vi "Test App Remove Process.vi"(8 "error in (no error)":errorcluster, 11 "Rig Test in":refnum<class "Application Test.lvclass">) -> (0 "error out":errorcluster, 3 "Rig Test out":refnum<class "Application Test.lvclass">)   [LabVIEW 2020, in "Application Test.lvclass"]
uses:
  Application Test.lvclass
  C:/Program Files (x86)/National Instruments/LabVIEW 2020/vi.lib/Astemes/LUnit/Test Case.lvclass
  Framework/Process/Process.lvclass
  Framework/Process/Process.lvclass/Process.ctl
  Framework/Application/Application.lvclass/Application.ctl
  <vilib>/Astemes/LUnit/Test Case.lvclass/Test Case.ctl
  <vilib>/Astemes/LUnit/LUnit Assertion Result.lvclass/LUnit Assertion Result.ctl
  <vilib>/Astemes/LUnit/LUnit Test Case Result.lvclass/LUnit Test Case Result.ctl
  <vilib>/Astemes/LUnit/LUnit Method Result.lvclass/LUnit Method Result.ctl
  Framework/Process/Public/Lifecycle/Get Lifecycle State.vi
  Framework/Process/Protected/Messaging/Request Message.vi
  Framework/Application/Private/Add Process to Map.vi
  Framework/Application/Private/Start Idle Processes if Running.vi
  Framework/Application/Private/Throw Error If Process Already in App.vi
  Framework/Process/Protected/Messaging/Enqueue Message.vi
  Framework/Process/Protected/SubVIs/Set Context.vi
  Framework/Application/Private/Remove Process from App.vi
  Framework/Application/Private/Parse Process Name.vi
  Framework/Application/Private/Remove Process from Map.vi
  Framework/Process/Protected/SubVIs/Clear Context.vi
  <vilib>/Astemes/LUnit/Palette/Pass If Equal.vi/cbf50e99-f124-4847-863a-8e9794d3dede.vi
  Framework/Process/Private/SubVIs/Wait for finish.vi
  Framework/Process/Private/SubVIs/Set Lifecycle State.vi
  <vilib>/Utility/error.llb/Clear Errors.vi
  Framework/Process/Private/SubVIs/Handle Debug Data.vi
  Framework/Process/Private/SubVIs/Enqueue Request Message.vi
  Framework/Application/Public/Get Process.vi
  Framework/Process/Public/Lifecycle/Leave Process Loop.vi
  <vilib>/AdvancedString/Delimited String to 1D String Array.vi
  <vilib>/Astemes/LUnit/Palette/Pass.vi
  <vilib>/Astemes/LUnit/Palette/Fail.vi
  <vilib>/Astemes/LUnit/Compare Variants.vi
  <vilib>/Astemes/LUnit/Describe Comparison.vi
  <vilib>/Astemes/LUnit/Set Assertion Type.vi
  Framework/Logging/Log Debug.vi
  <vilib>/AdvancedString/1D String Array to Delimited String.vi
  <vilib>/Utility/High Resolution Relative Seconds.vi
  Framework/Application/Private/Retrieve Process from App.vi
  Framework/Application/Private/Get Process from Map.vi
  <vilib>/Astemes/LUnit/Add test result.vi
  <vilib>/Astemes/LUnit/LUnit Write Passed.vi
  <vilib>/Astemes/LUnit/LUnit Write Message.vi
  <vilib>/Astemes/LUnit/LUnit Write Description.vi
  <vilib>/Astemes/LUnit/Variant to string.vi
  <vilib>/Astemes/LUnit/LUnit Write Assertion Type.vi
  <vilib>/Astemes/LUnit/LUnit Record Assertion Result.vi
  <vilib>/Astemes/LUnit/LUnit Aggregate Assertion Results.vi
  <vilib>/Astemes/LUnit/Assertion Result/LUnit Read Status.vi
  <vilib>/Astemes/LUnit/LUnit Read Message.vi
  <vilib>/Astemes/LUnit/LUnit Read Description.vi
  <vilib>/Astemes/LUnit/Method Result/LUnit Merge Status.vi
  <vilib>/Astemes/LUnit/LUnit Concatenate result strings.vi
  Framework/Application/Application.lvclass
  C:/Git/astemes-triarc-framework/source/Framework/Process/Process.lvclass
  <vilib>/Utility/error.llb/Error Cluster From Error Code.vi
  Framework/Process/Public/Read Name.vi
  Framework/Process/Private/SubVIs/Wait for Response Message.vi
  <vilib>/Utility/Data Type/Get Type Information.vi
  <vilib>/Utility/LVClass/Get LV Class Name.vi
  <vilib>/Astemes/LUnit/LUnit Assertion Result.lvclass
  Application Test.lvclass/Application Test.ctl
  <vilib>/Astemes/LUnit/Test Case.lvclass
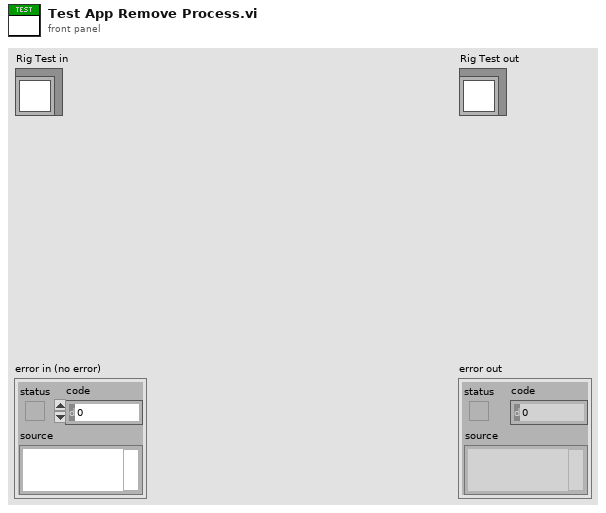
[diagram p1: front panel]
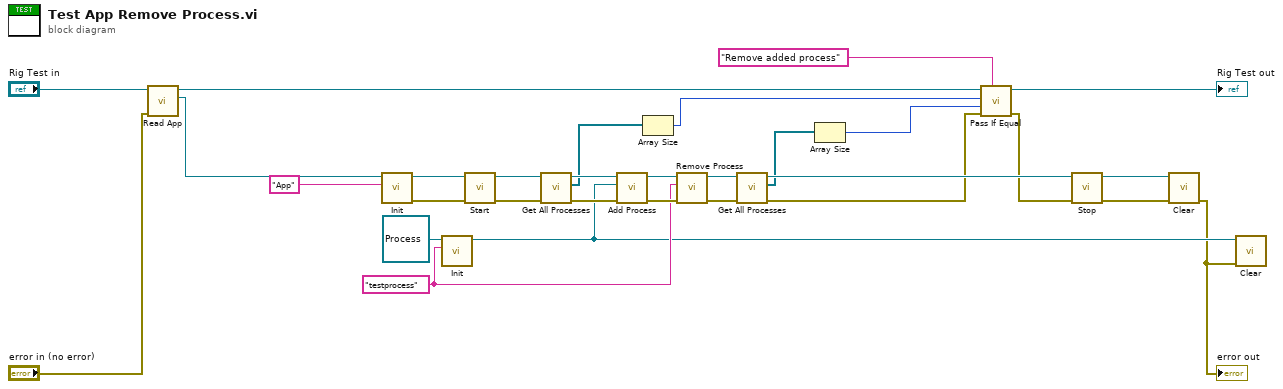
[diagram p0: block diagram]
diagram:
  w3 = "testprocess" ("Name")
  n1 = call "Read App.vi"("error in (no error)"="error in (no error)", "Application Test In"="Rig Test in") -> ("App out"=w29:refnum<class "Application.lvclass">, "Application Test Out"=w18:refnum<class "Application Test.lvclass">)  [unwired: 7 in, 1 out]
  n2 = call-dynamic "Init.vi"("Name"="App", "Process In"=w29) -> ("error out"=w19:errorcluster, "Process Out"=w20:refnum<class "Application.lvclass">)  [unwired: 8 in]
  n3 = call-dynamic "Init.vi"("Name"=w3, "Process In"=refnum<class "Process.lvclass"> refnum ("Process.lvclass")) -> ("Process Out"=w2:refnum<class "Process.lvclass">)  [unwired: 8 in, 1 out]
  n4 = call "Start.vi"("error in (no error)"=w19, "Process In"=w20) -> ("error out"=w21:errorcluster, "Process Out"=w7:refnum<class "Application.lvclass">)  [unwired: 7 in, 1 out]
  n5 = call "Get All Processes.vi"("error in (no error)"=w21, "Application In"=w7) -> ("error out"=w8:errorcluster, "App Processes"=w4:refnum<class "Process.lvclass">[], "Application Out"=w6:refnum<class "Application.lvclass">)  [unwired: 7 in]
  n6 = call "Add Process.vi"("error in (no error)"=w8, "Process"=w2, "Application In"=w6) -> ("error out"=w25:errorcluster, "Application Out"=w13:refnum<class "Application.lvclass">)  [unwired: 7 in]
  n7 = Array Size(array=w4) -> (size(s)=w5:i32)
  n8 = call "Remove Process.vi"("error in (no error)"=w25, "Process Name"=w3, "Application In"=w13) -> ("error out"=w14:errorcluster, "Application Out"=w12:refnum<class "Application.lvclass">)  [unwired: 6 in, 1 out]
  n9 = call "Get All Processes.vi"("error in (no error)"=w14, "Application In"=w12) -> ("error out"=w11:errorcluster, "App Processes"=w10:refnum<class "Process.lvclass">[], "Application Out"=w27:refnum<class "Application.lvclass">)  [unwired: 7 in]
  n10 = Array Size(array=w10) -> (size(s)=w9:i32)
  n11 = call <vilib>:"Pass If Equal.vi"("Description"="Remove added process", "error in (no error)"=w11, "Actual"=w9, "Expected"=w5, "LUnit Test Case In"=w18) -> ("error out"=w23:errorcluster, "LUnit Test Case Out"=→"Rig Test out":refnum<class "Application Test.lvclass">)  [unwired: 5 in]
  n12 = call "Stop.vi"("error in (no error)"=w23, "Process In"=w27) -> ("error out"=w16:errorcluster, "Process Out"=w15:refnum<class "Application.lvclass">)  [unwired: 7 in, 1 out]
  n13 = call-dynamic "Clear.vi"("error in (no error)"=w16, "Application In"=w15) -> ("error out"=w1:errorcluster)  [unwired: 9 in]
  "error out" <- w1
  n14 = call-dynamic "Clear.vi"("error in (no error)"=w1, "Process In"=w2) -> ()  [unwired: 9 in, 1 out]
